vi "Create Text Icon.vi"(8 "error in (no error)":errorcluster, 10 "Icon Text String":string, 11 "VI in":refnum<vi>) -> (0 "error out":errorcluster, 3 "VI out":refnum<vi>)   [LabVIEW 2020, in "Method Generation.lvlib" / "Support.lvlib"]
uses:
  Support.lvlib
  <vilib>/LabVIEW Icon API/LabVIEW Icon API.lvlib
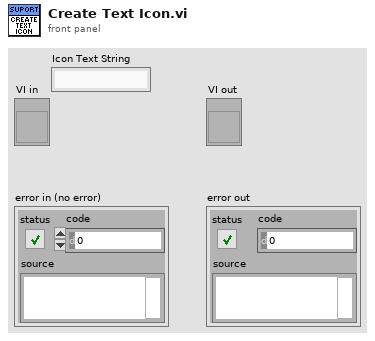
[diagram p1: front panel]
types:
  T1 = cluster{"[0]":string, "[1]":string, "[2]":string, "[3]":string}
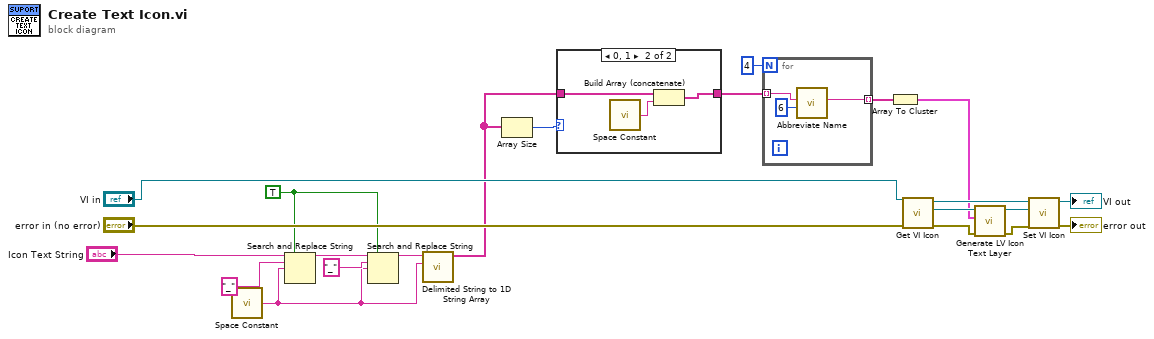
[diagram p0: block diagram]
diagram:
  w17 = TRUE
  n1 = call <vilib>:"Space Constant.vi"() -> ("String"=w14:string)
  n2 = Search and Replace String(replace all?=w17, input string="Icon Text String", search string="_", replace string=w14) -> (result string=w18:string)  [unwired: 4 in, 3 out]
  n3 = Search and Replace String(replace all?=w17, input string=w18, search string="_", replace string=w14) -> (result string=w13:string)  [unwired: 4 in, 3 out]
  n4 = call <vilib>:"Delimited String to 1D String Array.vi"("delimiter"=w14, "delimited string"=w13) -> ("string array"=w2:string[])  [unwired: 9 in]
  n5 = Array Size(array=w2) -> (size(s)=w3:i32)
  n6 = case shown="0, 1" w3 {
    tunnel: w2 -> [w23 w25]
    tunnel: [w23 w24] -> w1
    frame Default {
    }
    frame 0, 1 {
      n7 = call <vilib>:"Space Constant.vi"() -> ("String"=w26:string)
      n8 = Build Array (concatenate)(w25, w26) -> (w24:string[])
    }
  }
  n9 = for {
    N: 4 -> [_]
    tunnel: w1 -> [w28] mode=indexing
    tunnel: [w27] -> w7 mode=indexing
    n10 = call "Abbreviate Name.vi"("Max Length"=6, "Long Name"=w28) -> ("Abreviated Name"=w27:string)  [unwired: 8 in, 1 out]
  }
  n11 = Array To Cluster(array=w7) -> (cluster=w6:T1)
  n12 = call <vilib>:"Get VI Icon.vi"("error in (no error)"="error in (no error)", "VI Refnum in"="VI in") -> ("error out"=w9:errorcluster, "Icon"=w10:refnum<class "Icon.lvclass">, "VI Refnum out"=w11:refnum<vi>)  [unwired: 7 in]
  n13 = call <vilib>:"Generate LV Icon Text Layer.vi"("error in (no error)"=w9, "Text"=w6, "Icon in"=w10) -> ("error out"=w8:errorcluster, "Icon out"=w22:refnum<class "Icon.lvclass">)  [unwired: 7 in]
  n14 = call <vilib>:"Set VI Icon.vi"("error in (no error)"=w8, "Icon"=w22, "VI Refnum in"=w11) -> ("error out"=→"error out":errorcluster, "VI Refnum out"=→"VI out":refnum<vi>)  [unwired: 7 in]
